vi "CheckNewCMD.vi"(8 "DeviceIndex":i32, 11 "MB_CMD_In":T1[](array[typedef]) {"Function Code" items=["Read Coils"=1, "Read Discrete Inputs"=2, "Read Holding Registers"=3, "Read Input Registers"=4, "Write Single Coil"=5, "Write Single Register"=6, "Read Exception Status"=7, "Write Multiple Coils"=15, "Write Multiple Registers"=16]}) -> (3 "MB_CMD_Out":T1[](array[typedef]) {"Function Code" items=["Read Coils"=1, "Read Discrete Inputs"=2, "Read Holding Registers"=3, "Read Input Registers"=4, "Write Single Coil"=5, "Write Single Register"=6, "Read Exception Status"=7, "Write Multiple Coils"=15, "Write Multiple Registers"=16]})   [LabVIEW 2020, in "ModBusCommon.lvlib"]
uses:
  ModBusCommon.lvlib
  DriverCommon/MB Modbus Command.ctl
  DynamicIOCMD.lvlib
  DriverCommon.lvlib
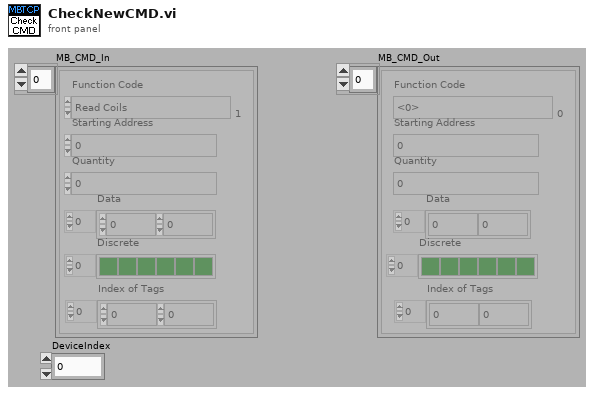
[diagram p1: front panel]
types:
  T1 = typedef "DriverCommon.lvlib/MB Modbus Command.ctl" = cluster{"Function Code":u8, "Starting Address":u16, "Quantity":u16, "Data":u16[], "Discrete":bool[], "Index of Tags":i32[]}
  T2 = typedef "DynamicIOCMD.lvlib/DynamicIOCMD.ctl" = cluster{"Data":dbl, "Register":string, "DataType":string, "Address":string, "Protocol":string, "IOAddress":cluster{"Register":i32, "Address":i32, "Device":i32, "Length":i32, "Offset":i32}, "WriteMode":string}
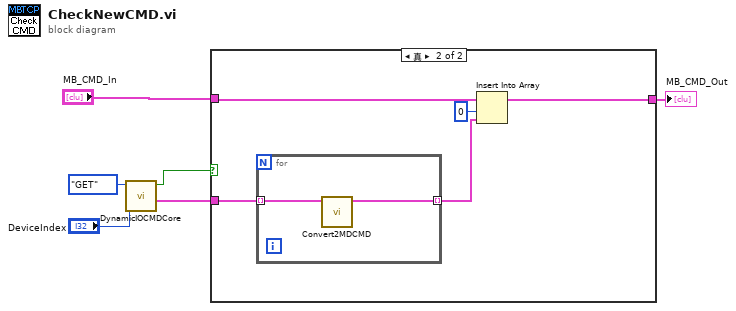
[diagram p0: block diagram]
diagram:
  n1 = call "DynamicIOCMDCore.vi"("DeviceIndex"="DeviceIndex", "Function"=enum16{"INIT", "NEW", "GET"}."GET") -> ("NewCMD"=w2:T2[], "Have new write CMD"=w4:bool)  [unwired: 8 in]
  n2 = case shown="真" w4 {
    tunnel: "MB_CMD_In" -> [w7 w11]
    tunnel: w2 -> [_ w12]
    tunnel: [w7 w8] -> w1
    frame False {
    }
    frame True {
      n3 = for {
        tunnel: w12 -> [w14] mode=indexing
        tunnel: [w13] -> w9 mode=indexing
        n4 = call "Convert2MDCMD.vi"("New_Write_CMD"=w14) -> ("MBWriteCMD"=w13:T1)  [unwired: 10 in]
      }
      n5 = Insert Into Array(array=w11, index=0, new element=w9) -> (w8:T1[])
    }
  }
  "MB_CMD_Out" <- w1
